vi "Set SpecimenTempCtrlSettings.vi"(4 "Lower deviation":dbl, 6 "Upper deviation":dbl, 7 "Ctrl Status (On/Off)":bool, 8 "error in (no error)":errorcluster, 10 "Address (0)":i32, 11 "VISA resource name":refnum<visa-resource-name>) -> (0 "error out":errorcluster, 3 "VISA resource name out":refnum<visa-resource-name>)   [LabVIEW 2021, in "Environment Chamber.lvlib" / "Climatic Chamber.lvlib"]
doc: "<b>Constant setup specimen temperature settings</B>\n\nSets the specimen temperature control set point, the upper deviation and lower dviation in constant setup."
uses:
  Climatic Chamber.lvlib
panel:
  out "NACK":bool
  out "Error":bool
  out "ACK":bool
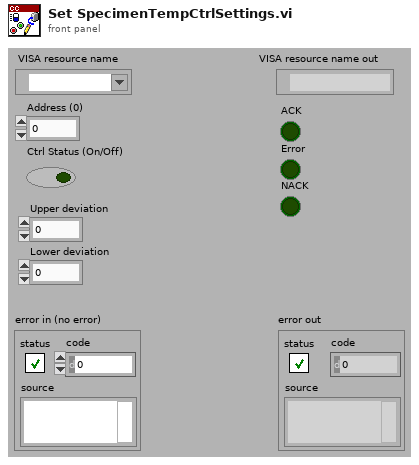
[diagram p1: front panel]
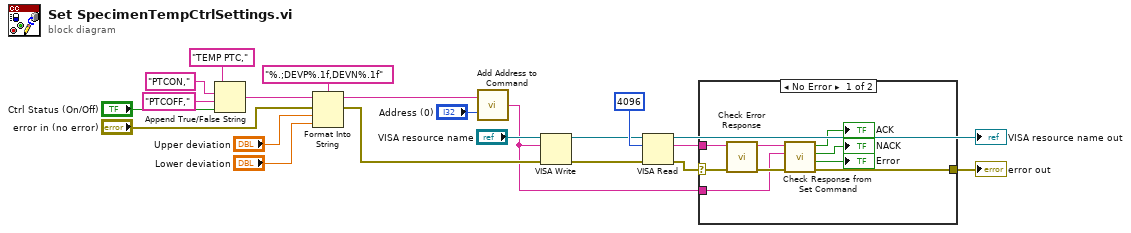
[diagram p0: block diagram]
diagram:
  n1 = Append True/False String(1:"Ctrl Status (On/Off)", 2:"PTCOFF," ("true string"), 3:"PTCON," ("true string"), 4:"TEMP PTC,") -> (0:w6:string)
  n2 = Format Into String(format string="%.;DEVP%.1f,DEVN%.1f", initial string=w6, error in="error in (no error)", "Upper deviation", "Lower deviation") -> (resulting string=w1:string, error out=w21:errorcluster)
  n3 = call "Add Address to Command.vi"("Address (0)"="Address (0)", "Command"=w1) -> ("Command OUT"=w11:string)
  n4 = VISA Write(VISA resource name="VISA resource name", write buffer=w11, error in (no error)=w21) -> (VISA resource name out=w18:refnum<visa-resource-name>, error out=w17:errorcluster)  [unwired: 1 out]
  n5 = VISA Read(VISA resource name=w18, byte count=u32 4096, error in (no error)=w17) -> (VISA resource name out=→"VISA resource name out":refnum<visa-resource-name>, read buffer=w13:string, error out=w14:errorcluster)  [unwired: 1 out]
  n6 = case shown="No Error" w14 {
    selector: w14 -> [w29 w31]
    tunnel: w13 -> [w30 _]
    tunnel: [w25 w31] -> w12
    tunnel: w11 -> [w26 _]
    frame No Error {
      n7 = call "Check Error Response.vi"("error in (no error)"=w29, "read String"=w30) -> ("error out"=w28:errorcluster, "String out"=w27:string)  [unwired: 7 in, 1 out]
      n8 = call "Check Response from Set Command.vi"("error in (no error)"=w28, "Command"=w26, "Response"=w27) -> ("error out"=w25:errorcluster, "Error"=→"Error":bool, "NACK"=→"NACK":bool, "ACK"=→"ACK":bool)  [unwired: 5 in]
    }
    frame Error {
    }
  }
  "error out" <- w12
